vi "ex_sortOutManualAndAutoFillProperties.vi"(5 "User-defined properties":T1[](array[typedef])) -> (0 "channelgroup props":T4[](array[typedef]), 1 "channel props":T4[](array[typedef]), 2 "file props":T4[](array[typedef]), 3 "property names (manual)":string[](array[string]), 4 "property names (autofill)":string[](array[string]))   [LabVIEW 2017]
uses:
  <vilib>/express/express shared/ExFile.llb/ex_TdmProperty.ctl
  <vilib>/express/express shared/ex_EditUserDefinedProperties/usiDataType.ctl
  <vilib>/express/express shared/ExFile.llb/ex_userDefProperty.ctl
  <vilib>/express/express shared/ExFile.llb/ex_propertySource.ctl
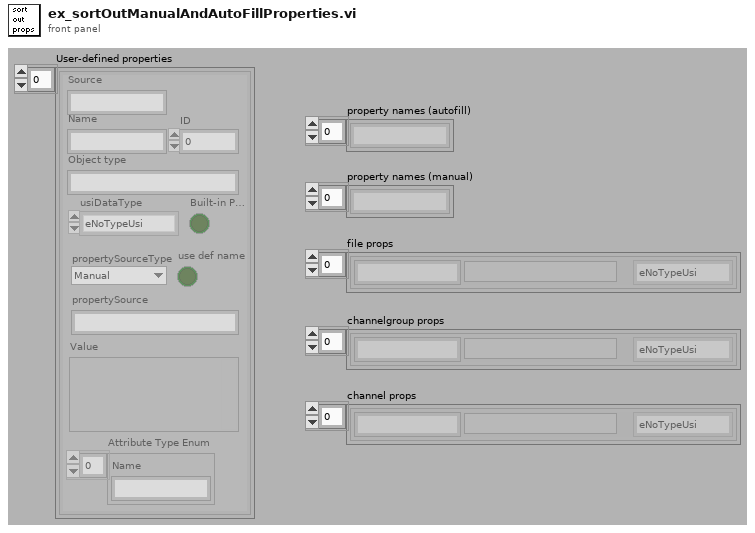
[diagram p1: front panel]
types:
  T1 = typedef "ex_userDefProperty.ctl" = cluster{"Name":string, "Object type":string, "usiDataType":T2, "propertySourceType":T3, "propertySource":string, "Value":variant, "ID":i32, "use def name":bool, "Source":string, "Built-in Prop":bool, "Attribute Type Enum":string[]}
  T2 = typedef "usiDataType.ctl" = enum16{"eNoTypeUsi", "eInt8Usi", "eInt16Usi", "eInt32Usi", "eInt64Usi", "eUInt8Usi", "eUInt16Usi", "eUInt32Usi", "eUInt64Usi", "eFloat32Usi", "eFloat64Usi", "- 0", "- 1", "- 2", "- 3", "- 4", "- 5", "- 6", "- 7", "- 8", "- 9", "eString8Usi", "eString16Usi", "eStringUsi", "eEnumUsi", "- 10", "- 11", "- 12", "- 13", "- 14", "eTimeUsi", "- 15", "- 16", "- 17", "- 18", "- 19", "- 20", "- 21", "- 22", "- 23", "eInstanceUsi", "eStoreUsi"}
  T3 = typedef "ex_propertySource.ctl" = enum16{"Manual", "System", "DAQmx Channel", "Terminal", "Ignore"}
  T4 = typedef "ex_TdmProperty.ctl" = cluster{"Name":string, "Type":T2, "Value":variant}
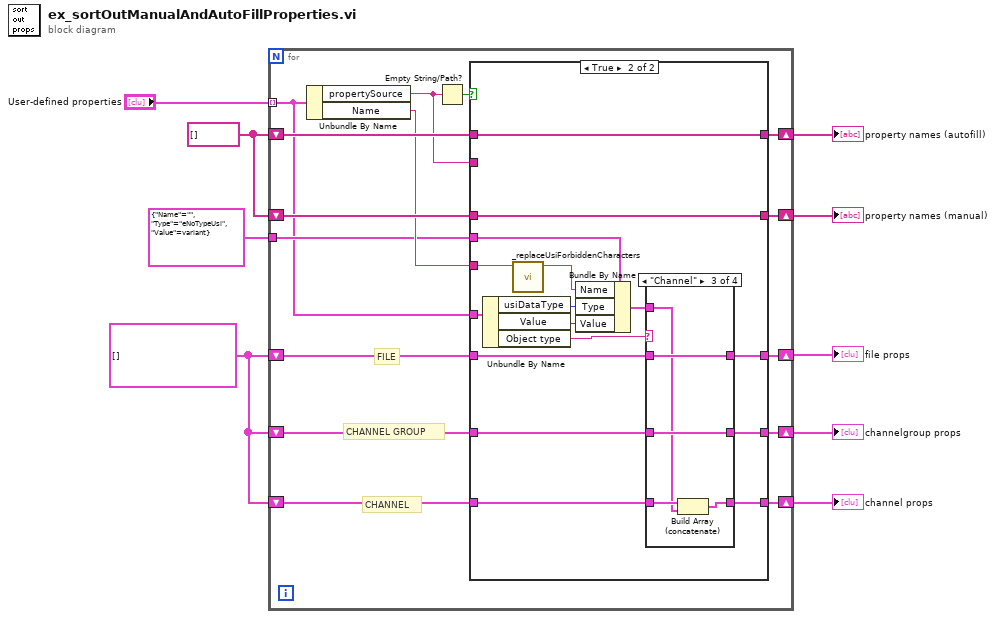
[diagram p0: block diagram]
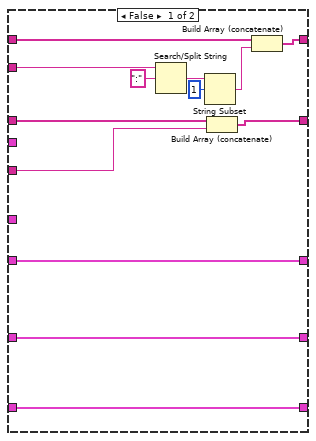
[diagram p2: hidden frame]
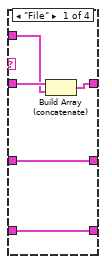
[diagram p3: hidden frame]
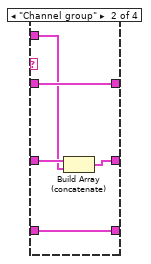
[diagram p4: hidden frame]
diagram:
  w6 = T4[] []
  w2 = string[] []
  n1 = for {
    tunnel: "User-defined properties" -> [w14] mode=indexing
    shift-right: [w23] -> w4
    shift-left: w2 -> [w24]
    shift-right: [w21] -> w3
    shift-left: w2 -> [w20]
    shift-right: [w16] -> w8
    shift-left: w6 -> [w17]
    tunnel: T4 {"Name"="", "Type"=enum."eNoTypeUsi", "Value"=variant} ("TDM Property") -> [w15]
    shift-right: [w13] -> w9
    shift-left: w6 -> [w12]
    shift-right: [w10] -> w7
    shift-left: w6 -> [w11]
    # "CHANNEL"
    # "CHANNEL GROUP"
    # "FILE"
    n2 = Unbundle By Name(w14) -> ("propertySource"=w19:string, "Name"=w18:string)
    n3 = Empty String/Path?(string/path=w19) -> (empty?=w22:bool)
    n4 = case shown="True" w22 {
      tunnel: w24 -> [w37 w53]
      tunnel: [w36 w53] -> w23
      tunnel: w20 -> [w33 w52]
      tunnel: [w34 w52] -> w21
      tunnel: w18 -> [w35 w39]
      tunnel: w19 -> [w32 _]
      tunnel: w17 -> [w27 w47]
      tunnel: [w27 w46] -> w16
      tunnel: w15 -> [_ w51]
      tunnel: w14 -> [_ w50]
      tunnel: w12 -> [w26 w43]
      tunnel: [w26 w44] -> w13
      tunnel: w11 -> [w25 w42]
      tunnel: [w25 w41] -> w10
      frame False {
        n5 = Search/Split String(string=w32, search string/char (-)=":") -> (match + rest of string=w30:string)  [unwired: 1 in, 2 out]
        n6 = String Subset(string=w30, offset (0)=1) -> (substring=w28:string)  [unwired: 1 in]
        n7 = Build Array (concatenate)(w33, w35) -> (w34:string[])
        n8 = Build Array (concatenate)(w37, w28) -> (w36:string[])
      }
      frame True {
        n9 = Unbundle By Name(w50) -> ("usiDataType"=w48:T2, "Value"=w49:variant, "Object type"=w40:string)
        n10 = call <vilib>:"_replaceUsiForbiddenCharacters.vi"("string in"=w39) -> ("string out"=w38:string)  [unwired: 5 in, 1 out]
        n11 = Bundle By Name(cluster=w51, "Name"=w38, "Type"=w48, "Value"=w49) -> (w45:T4)
        n12 = case shown="\"Channel\"" w40 {
          tunnel: w47 -> [w58 w61 w65 w70]
          tunnel: [w57 w61 w65 w70] -> w46
          tunnel: w45 -> [w56 w59 w64 _]
          tunnel: [w55 w63 w66 w71] -> w44
          tunnel: w43 -> [w55 w62 w66 w71]
          tunnel: w42 -> [w54 w60 w68 w69]
          tunnel: [w54 w60 w67 w69] -> w41
          frame "File" {
            n13 = Build Array (concatenate)(w58, w56) -> (w57:T4[])
          }
          frame "Channel group" {
            n14 = Build Array (concatenate)(w62, w59) -> (w63:T4[])
          }
          frame "Channel" {
            n15 = Build Array (concatenate)(w68, w64) -> (w67:T4[])
          }
          frame Default {
          }
        }
      }
    }
  }
  "channelgroup props" <- w9
  "file props" <- w8
  "channel props" <- w7
  "property names (autofill)" <- w4
  "property names (manual)" <- w3
